vi "util.proc.set-name.vi"(8 "error in":errorcluster, 10 "new Proc Name":string, 11 "Procedure in":variant[](array[variant])) -> (0 "error out":errorcluster, 3 "Procedure out":variant[](array[variant]))   [LabVIEW 2024]
uses:
  controls/typeProcVarientName.ctl
  Polymorphics/variantCtrlString.vi
  proc.util.validateParamExist.vi
  <vilib>/Utility/error.llb/Clear Errors.vi
  util.error.create.vi
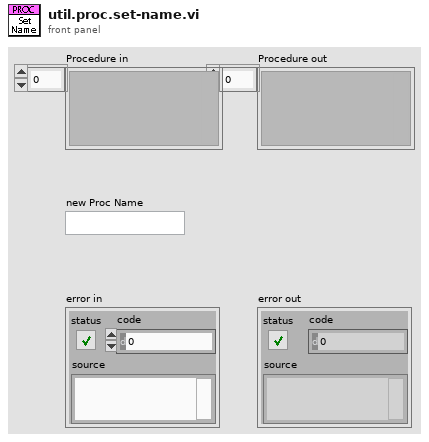
[diagram p1: front panel]
types:
  T1 = typedef "typeProcVarientName.ctl" = enum16{"procNameID", "procModuleID", "procPath", "procIsRunning", "procIndex", "procModule", "procRegisterNumeric", "procRegisterString", "procReport", "procReportPrev", "procCLK", "procStepPointer", "procType"}
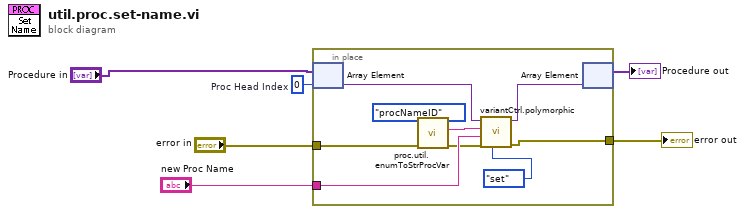
[diagram p0: block diagram]
diagram:
  w6 = 0  # Proc Head Index
  n1 = in-place {
    in-place-border: "new Proc Name" -> [w11]
    in-place-border: "error in" -> [w10]
    in-place-border: [w9] -> w1
    n2 = in-place-array #1("Procedure in", w6) -> (w8:variant)
    n3 = call "proc.util.enumToStrProcVar.vi"("Proc var"=typeProcVarientName."procNameID" ("Combo Box")) -> ("String"=w14:string)  [unwired: 10 in]
    n4 = call-poly "variantCtrl.polymorphic.vi"("menu in (get)"=enum16{"get", "set"}."set", "error in"=w10, "String Value"=w11, "name in"=w14, "Step in"=w8) -> ("error out"=w9:errorcluster, "Step out"=w7:variant)  [unwired: 3 in, 2 out]
    n5 = in-place-array #1(w7) -> (→"Procedure out":variant[])  [unwired: 1 out]
  }
  "error out" <- w1
